vi "Nctp Ramp Running.vi"(4 "Close Received":bool, 5 "MCL Ramp Running?":bool, 6 "error in":errorcluster, 7 "Stop Requests":T1, 9 "MCL Cmd In":refnum<queue>) -> (0 "error out":errorcluster, 2 "NTCP MM Finish State":T2, 3 "MCL Cmd Out":refnum<queue>)   [LabVIEW 2009]
uses:
  NTCP Client/MM 2 NTCP Message.ctl
  NTCP library/NTCP Commands.ctl
  Apps/Yes No Button.ctl
  NTCP Mixed Mode States.ctl
  Stop Requests.ctl
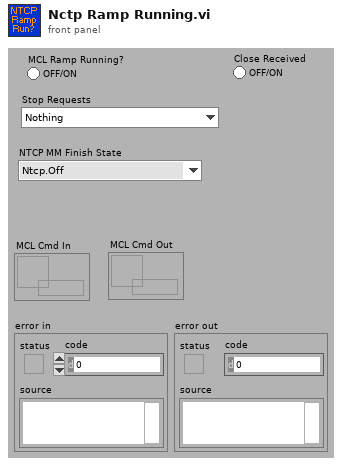
[diagram p1: front panel]
types:
  T1 = typedef "Stop Requests.ctl" = enum16{"Nothing", "Stop Requested", "Abort Requested"}
  T2 = typedef "NTCP Mixed Mode States.ctl" = enum16{"Ntcp.Off", "Ntcp.WaitForProposal", "Ntcp.WaitForAccept", "Ntcp.WaitForExecute", "Ntcp.WaitForStart", "Ntcp.WaitForMclRamp", "Ntcp.WaitForMclDone", "Ntcp.Shutdown"}
  T3 = typedef "MM 2 NTCP Message.ctl" = cluster{"NTCP commands":T4, "Transaction ID":string, "Control Point":string, "Accepted":T5}
  T4 = typedef "NTCP Commands.ctl" = enum16{"propose", "execute", "cancel", "set-parameter", "get-parameter", "open-session", "close-session", "get-control-point", "Unknown", "stop"}
  T5 = typedef "Yes No Button.ctl" = bool
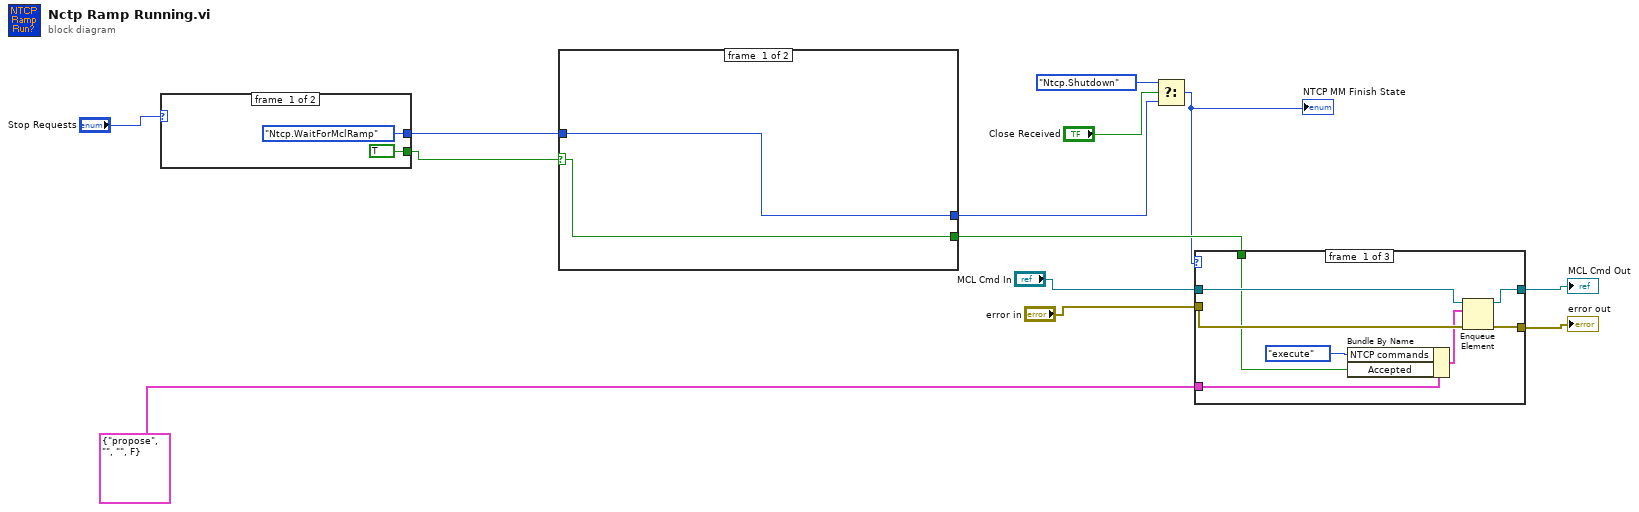
[diagram p0: block diagram]
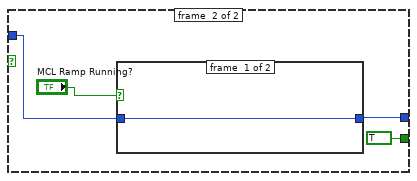
[diagram p2: hidden frame]
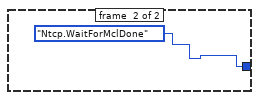
[diagram p3: hidden frame]
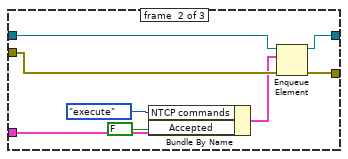
[diagram p4: hidden frame]
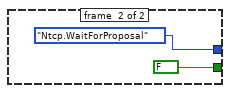
[diagram p6: hidden frame]
diagram:
  n1 = case shown="\"Nothing\"" "Stop Requests" {
    tunnel: [NTCP_Mixed_Mode_States."Ntcp.WaitForMclRamp" ("NTCP MM States") NTCP_Mixed_Mode_States."Ntcp.WaitForProposal" ("NTCP MM States")] -> w3
    tunnel: [TRUE FALSE] -> w1
    frame #0 {
    }
    frame #1 {
    }
  }
  n2 = case shown="True" w1 {
    selector: w1 -> [w19 _]
    tunnel: [w19 TRUE] -> w13
    tunnel: [w18 w20] -> w4
    tunnel: w3 -> [w18 w22]
    frame #0 {
    }
    frame #1 {
      n3 = case shown="False" "MCL Ramp Running?" {
        tunnel: [w24 NTCP_Mixed_Mode_States."Ntcp.WaitForMclDone" ("NTCP MM States")] -> w20
        tunnel: w22 -> [w24 _]
        frame #0 {
        }
        frame #1 {
        }
      }
    }
  }
  n4 = Select(t=NTCP_Mixed_Mode_States."Ntcp.Shutdown", s="Close Received", f=w4) -> (s? t:f=w7:T2)
  "NTCP MM Finish State" <- w7
  n5 = case shown="\"Ntcp.WaitForProposal\"" w7 {
    tunnel: T3 {"NTCP commands"=enum."propose", "Transaction ID"="", "Control Point"="", "Accepted"=FALSE} ("NTCP Message") -> [w33 w41 _]
    tunnel: "MCL Cmd In" -> [w31 w38 w43]
    tunnel: [w30 w37 w43] -> w10
    tunnel: "error in" -> [w29 w36 w42]
    tunnel: [w28 w35 w42] -> w12
    tunnel: w13 -> [w26 _ _]
    frame #0 {
      n6 = Bundle By Name(cluster=w33, "NTCP commands"=NTCP_Commands."execute", "Accepted"=w26) -> (w27:T3)
      n7 = Enqueue Element(queue=w31, element=w27, error in (no error)=w29) -> (queue out=w30:refnum<queue>, error out=w28:errorcluster)  [unwired: 1 in, 1 out]
    }
    frame #1 {
      n8 = Bundle By Name(cluster=w41, "NTCP commands"=NTCP_Commands."execute", "Accepted"=T5 FALSE) -> (w34:T3)
      n9 = Enqueue Element(queue=w38, element=w34, error in (no error)=w36) -> (queue out=w37:refnum<queue>, error out=w35:errorcluster)  [unwired: 1 in, 1 out]
    }
    frame #2 {
    }
  }
  "error out" <- w12
  "MCL Cmd Out" <- w10
